vi "SGL info.vi"(8 "error in (no error)":errorcluster, 11 "Variant":variant) -> (0 "error out":errorcluster, 3 "child strings":string[](array[string]))   [LabVIEW 2017, in "DSF Simple Explorer.lvlib"]
uses:
  DSF Configuration.llb/DSF Simple Explorer.lvlib
  DSF Configuration.llb/Get Numeric Information.vi
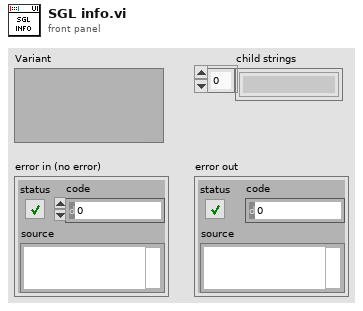
[diagram p1: front panel]
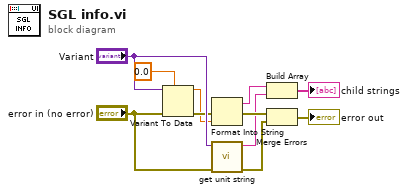
[diagram p0: block diagram]
diagram:
  n1 = Variant To Data(error in="error in (no error)", type=sgl 0.0, Variant="Variant") -> (data=w2:sgl, error out=w5:errorcluster)
  n2 = Format Into String(error in=w5, w2) -> (resulting string=w4:string, error out=w9:errorcluster)  [unwired: 2 in]
  n3 = call "get unit string.vi"("error in (no error)"="error in (no error)", "Variant"="Variant") -> ("error out"=w10:errorcluster, "String"=w8:string)  [unwired: 8 in]
  n4 = Build Array(w4, w8) -> (→"child strings":string[])
  n5 = Merge Errors(w9, w10) -> (→"error out":errorcluster)
